vi "Create Text Table.vi"(5 "Column Headers 2D [ ]":string[][](array[string]), 7 "Row Headers 1D [ ]":string[](array[string]), 9 "Text Data 2D [ ]":string[][](array[string])) -> (4 "Row Header?":bool, 6 "Header Column size":cluster{"# Column":u16, "# Row":u16}, 8 "Table size":cluster{"# Column":u16, "# Row":u16}, 10 "Text Table 2D [ ]":string[][](array[string]))   [LabVIEW 2019]
doc: "Developed by Jean-Marc Simard\nCopyright © 2012, Exaprom Inc.\nAll rights reserved.\nLicense: BSD\n\nWith iTextSharp 4.1.6 (http://itextsharp.sourceforge.net)\nunder Mozilla Public License Version 1.1\n(http://www.mozilla.org/MPL/MPL-1.1.html)"
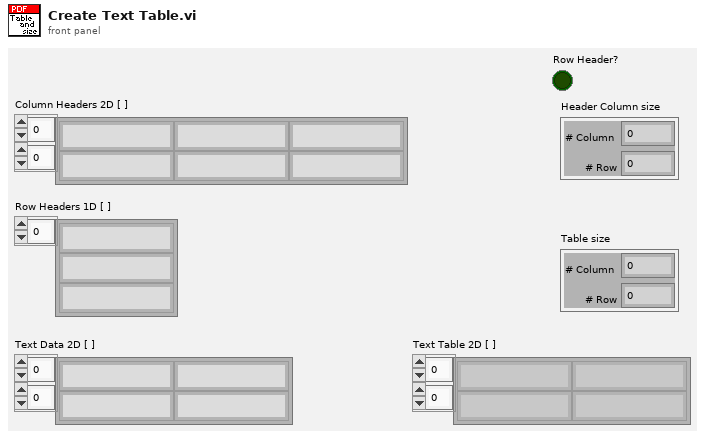
[diagram p1: front panel]
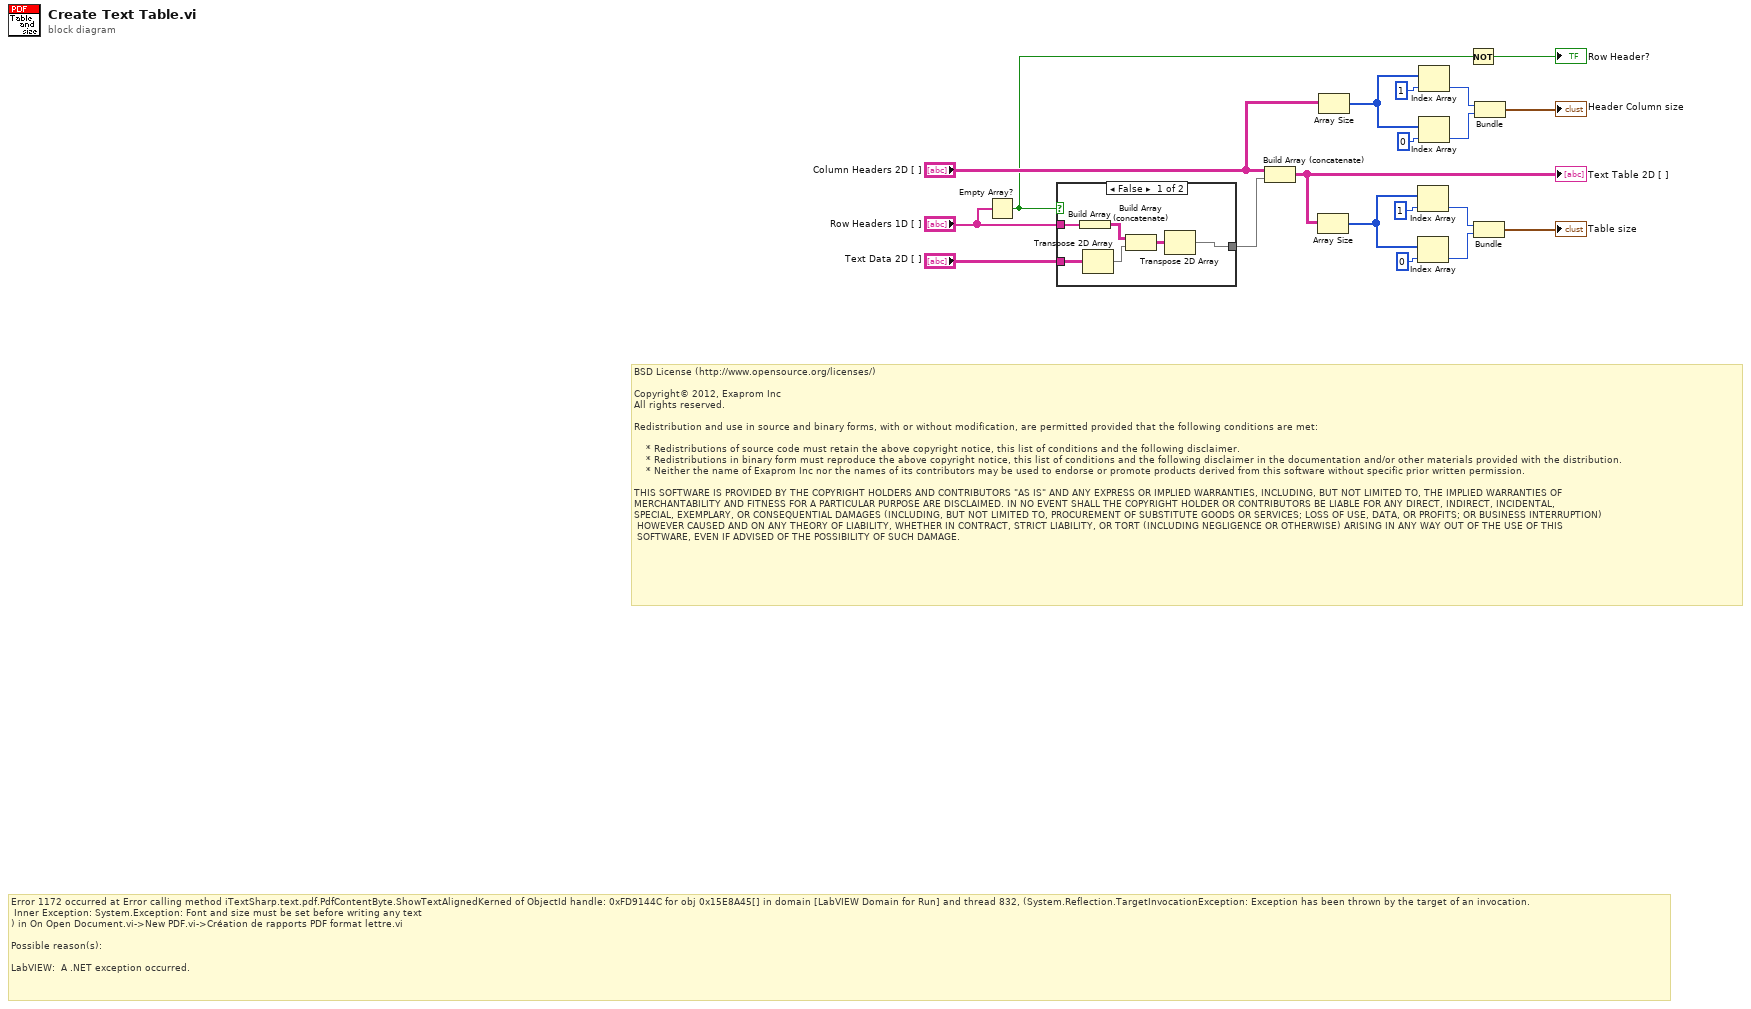
[diagram p0: block diagram]
diagram:
  # "Error 1172 occurred at Error calling method iTextSharp.text.pdf.PdfContentByte.ShowTextAlignedKerned of ObjectId handle: 0xFD9144C for obj 0x15E8A45[] in domain [LabVIEW Domain for Run] and thread 832, (System.Reflection.TargetInvocationException: Exception has been thrown by the target of an invocation.\n\tInner Exception: System.Exception: Font and size must be set before writing any text\n) in On Open Document.vi->New PDF.vi->Création de rapports PDF format lettre.vi\n\nPossible reason(s):\n\nLabVIEW:  A .NET exception occurred."
  # "BSD License (http://www.opensource.org/licenses/)\n\nCopyright© 2012, Exaprom Inc\nAll rights reserved.\n\nRedistribution and use in source and binary forms, with or without modification, are permitted provided that the following conditions are met:\n\n    * Redistributions of source code must retain the above copyright notice, this list of conditions and the following disclaimer.\n    * Redistributions in binary form must reproduce the above copyright notice, this list of conditions and the following disclaimer in the documentation and/or other materials provided with the distribution.\n    * Neither the name of Exaprom Inc nor the names of its contributors may be used to endorse or promote products derived from this software without specific prior written permission.\n\nTHIS SOFTWARE IS PROVIDED BY THE COPYRIGHT HOLDERS AND CONTRIBUTORS \"AS IS\" AND ANY EXPRESS OR IMPLIED WARRANTIES, INCLUDING, BUT NOT LIMITED TO, THE IMPLIED WARRANTIES OF \nMERCHANTABILITY AND FITNESS FOR A PARTICULAR PURPOSE ARE DISCLAIMED. IN NO EVENT SHALL THE COPYRIGHT HOLDER OR CONTRIBUTORS BE LIABLE FOR ANY DIRECT, INDIRECT, INCIDENTAL,\nSPECIAL, EXEMPLARY, OR CONSEQUENTIAL DAMAGES (INCLUDING, BUT NOT LIMITED TO, PROCUREMENT OF SUBSTITUTE GOODS OR SERVICES; LOSS OF USE, DATA, OR PROFITS; OR BUSINESS INTERRUPTION)\n HOWEVER CAUSED AND ON ANY THEORY OF LIABILITY, WHETHER IN CONTRACT, STRICT LIABILITY, OR TORT (INCLUDING NEGLIGENCE OR OTHERWISE) ARISING IN ANY WAY OUT OF THE USE OF THIS\n SOFTWARE, EVEN IF ADVISED OF THE POSSIBILITY OF SUCH DAMAGE."
  n1 = Empty Array?(array="Row Headers 1D [ ]") -> (empty?=w2:bool)
  n2 = case shown="False" w2 {
    tunnel: "Text Data 2D [ ]" -> [w23 w26]
    tunnel: [w20 w26] -> w18
    tunnel: "Row Headers 1D [ ]" -> [w25 _]
    frame False {
      n3 = Build Array(w25) -> (w21:string[][])
      n4 = Transpose 2D Array(2D array=w23) -> (transposed array=w22:string[][])
      n5 = Build Array (concatenate)(w21, w22) -> (w24:string[][])
      n6 = Transpose 2D Array(2D array=w24) -> (transposed array=w20:string[][])
    }
    frame True {
    }
  }
  n7 = Build Array (concatenate)("Column Headers 2D [ ]", w18) -> (w4:string[][])
  "Text Table 2D [ ]" <- w4
  n8 = Array Size(array=w4) -> (size(s)=w9:i32[])
  n9 = Array Size(array="Column Headers 2D [ ]") -> (size(s)=w15:i32[])
  n10 = Index Array(array=w9, index=1) -> (element=w6:i32)
  n11 = Index Array(array=w9, index=0) -> (element=w5:i32)
  n12 = Index Array(array=w15, index=1) -> (element=w12:i32)
  n13 = Index Array(array=w15, index=0) -> (element=w11:i32)
  n14 = Not(x=w2) -> (.not. x?=→"Row Header?":bool)
  n15 = Bundle(w6, w5) -> (→"Table size":cluster{i32, i32})  [unwired: 1 in]
  n16 = Bundle(w12, w11) -> (→"Header Column size":cluster{i32, i32})  [unwired: 1 in]
